vi "interface.vi"() -> ()   [LabVIEW 2019]
panel:
  out "alerte  2":bool=TRUE
  out "Error out 2":errorcluster
  out "marches _2":bool
  out "marche_one":bool
  out "alerte_high":bool
  out "alerte":bool
  out "type_sel":string
  out "concatenated string":string
  out ".not. x?":bool
  out "error out 4":errorcluster
  out "Error out":errorcluster
  in  "Add Square":bool
  in  "Database Square":bool
  in  "Dashboard Square":bool
  in  "Settings Square":bool
  in  "Tools Square":bool
  in  "Log Out Square":bool
  out "Log In Square":bool
  in  "Tab Control":enum32{"Page 1", "Page 2"}(tab)
  out "rouge":bool
  out "orange":bool
  out "vert":bool
  out "Historique des alertes":string
  in  "Tab Control 2":T1(tab)
  out "Boolean":bool
  in  "password":string
  in  "user name":string
  in  "Login Button":bool
  in  "Information Button":bool
  in  "type maintenace":bool
  in  "Energy 2":bool
  in  "Database Button":bool
  in  "Energy":bool
  in  "comp_2":bool
  in  "comp_1":bool
  in  "Tools Button":bool
  in  "autre maintenance":bool
  in  "Back Button":bool
  in  "compresseur id":dbl
  in  "Cluster 2":T2
  in  "Cluster":T3
  out "Derniére date de changement  H":string
  out "Nombre d'heure de marche H":string
  out "Durée de vie du huile":string
  out "Derniére date de changement C":string
  out "Nombre d'heure de marche C":string
  out "Durée de vie du courroie":string
  in  "autre maintenace bouton":bool
  in  "retour autre maintenace":bool
  in  "ID Comp":dbl
  in  "Commantaire":string
  in  "Description":string(combo)
  in  "Type maintenace":string(combo)
  out "error out 3":errorcluster
  in  "Back Square":bool
  out "error out 2":errorcluster
  in  "Url":string(combo)
  in  "Nom de la base":string(combo)
  in  "Back from 1":bool
  out "Debit":i32(knob) caption="Gauge" scale=0.0..80.0
  out "Etat":string
  out "Graphe de pression":cluster{timestamp[], dbl[]}(graph) caption="XY Graph - Dark"
  out "Graphe de Température":cluster{timestamp[], dbl[]}(graph) caption="XY Graph - Dark"
  out "Courant":i32(knob) caption="Gauge" scale=0.0..150.0
  out "Tension":i32(knob) caption="Gauge" scale=0.0..450.0
  out "Pression":i32(knob) caption="Gauge" scale=0.0..15.0
  out "Température":i32(knob) caption="Gauge" scale=0.0..150.0
  in  "Back from 2":bool
  out "Graphe de pression  2":cluster{timestamp[], dbl[]}(graph) caption="XY Graph - Dark"
  out "Graphe de Température":cluster{timestamp[], dbl[]}(graph) caption="XY Graph - Dark"
  out "Debit":i32(knob) caption="Gauge" scale=0.0..50.0
  out "Etat 2":string
  out "Courant  2":i32(knob) caption="Gauge" scale=0.0..150.0
  out "Tension 2":i32(knob) caption="Gauge" scale=0.0..250.0
  out "Pression 2":i32(knob) caption="Gauge" scale=0.0..10.0
  out "Température  2":i32(knob) caption="Gauge" scale=0.0..150.0
  out "COUT EN DT":dbl format="%_10g"
  in  "Prix KWH":string(combo)
  in  "Back from 3":bool
  in  "ID compresseur":dbl
  out "temp de marche en heure":dbl
  out "energie consommer kwh":dbl format="%_11g"
  in  "Date Fin":timestamp format="%<%.0X %x>T"
  in  "Date Debut":timestamp format="%<%.0X %x>T"
  out "Taux d’utilisation (%)":string
  out "Pression moyenne":string
  out "température moyenne":string
  out "Temps d'arret total":string
  in  "Back from 4":bool
  in  "ID compresseur":dbl
  out "Temps de fonctionnement total":string
  out "Nombre de démarrages / arrêts":string
  in  "Date Fin":timestamp format="%<%.0X %x>T"
  in  "Date Debut":timestamp format="%<%.0X %x>T"
  in  "Back Button 3":bool
  out "Historique des maintenances":string[][](table)
  out "Historique des alertes":string[][](table)
  in  "Back Button 4":bool
  in  "Add Button":bool
  in  "Role":string(combo)
  in  "Email":string
  in  "Mot de passe":string
  in  "Nom utilisateur":string
  in  "Back Button 2":bool
  in  "suivent":bool
  in  "TYPE C":bool
  in  "TYPE B":bool
  in  "type A":bool
  in  "Tab Control 3":enum32{"Page 1", "Page 2", "Page 3"}(tab)
  out "Nombre d'heures":dbl(slide)=1.0 scale=0.0..500.0
  out "Temps restants A":string
  out "Nombre d'heures":dbl(slide)=1.0 scale=0.0..1000.0
  out "Temps restants B":string
  out "Nombre d'heures":dbl(slide)=1.0 scale=0.0..4000.0
  out "Temps restants C":string
  in  "Temps de la maintenace":timestamp format="%<%H:%M>T"
  in  "Back Button 5":bool
  in  "Save Button":bool
  in  "Remarque":string
  in  "taches_principales":string
  in  "type_description":string(combo)
  in  "Type Maintenance":string(combo)
  out "Cluster - Thin Border 2":T4
  out "Cluster - Thin Border":T4
  in  "Back Button 6":bool
  # "Menu principale"
  # "Autre Maintenance"
  # "Paramètres"
  # "Controle énergie"
  # "kpi Performance"
  # "Historique"
  # "ajouter user"
  # "Maintenance type A :"
  # "Maintenance légère (préventive rapide)\nTâches à réaliser :\n\n-Vérification visuelle générale de la machine (fuites d’air, bruits anormaux).\n-Contrôle du niveau et de la qualité de l’huile.\n-Vidange de l’huile (si nécessaire selon le type d’huile).\n-Nettoyage des filtres d’aspiration d’air.\n-Inpection des courroies (tension et usure).\n-Contrôle de la température de fonctionnement.\n-Vérification des voyants d’alerte ou codes erreurs sur le pupitre."
  # "Maintenance type B :"
  # "Maintenance intermédiaire (préventive approfondie)\nTâches à réaliser :\n\n-Remplacement des courroies (même si elles ne semblent pas endommagées).\n-Remplacement systématique de l’huile du compresseur.\n-Nettoyage ou remplacement du filtre à air.\n-Nettoyage du refroidisseur (radiateur) pour éviter la surchauffe.\n-Vérification de la consommation électrique pour détecter les anomalies.\n-Contrôle du moteur électrique (bruit, vibrations, température)."
  # "Maintenance type C :"
  # "Maintenance lourde (grande révision)\nTâches à réaliser :\n\n-Remplacement des roulements du moteur et du compresseur.\n-Contrôle précis de l’étanchéité de tout le circuit d’air.\n-Recalibrage des capteurs de pression et de température.\n-Contrôle des soupapes (entrée/sortie) et nettoyage ou remplacement.\n-Inspection complète de la vis de compression (si applicable)."
  # "Info"
  # "Champ                                                           Valeur"
  # "Champ                                                           Valeur"
types:
  T1 = enum32{"Page 1", "Page 2", "Page 3", "Page 4", "Page 5", "Page 6", "Page 7", "Page 8", "Page 11", "Page 9", "Page 10", "Page 12", "Page 13", "Page 14"}
  T2 = cluster{"Save Button":bool, "Durée de vie huile ":dbl, "Description ":string, "Commantaire":string}
  T3 = cluster{"Save Button":bool, "Durée de vie courroie ":dbl, "Description ":string, "Commantaire":string}
  T4 = cluster{"Nom du compresseur":string, "Numéro de série\t":string, "Modèle\t":string, "Date de mise en service\t":string, "État actuel\t":string, "Heures de fonctionnement\t":string}
  T5 = enum32{"Page 1", "Page 2", "Page 3", "Page 4", "Page 5", "Page 6", "Page 7", "Page 8", "Page 11", "Page 9", "Page 10"}
  T6 = enum8{"Enabled", "Disabled", "Disabled and Grayed Out"}
  T7 = enum32{"Page 1", "Page 2", "Page 3", "Page 4", "Page 5", "Page 6", "Page 7", "Page 8", "Page 11", "Page 9", "Page 10", "Page 12", "Page 13"}
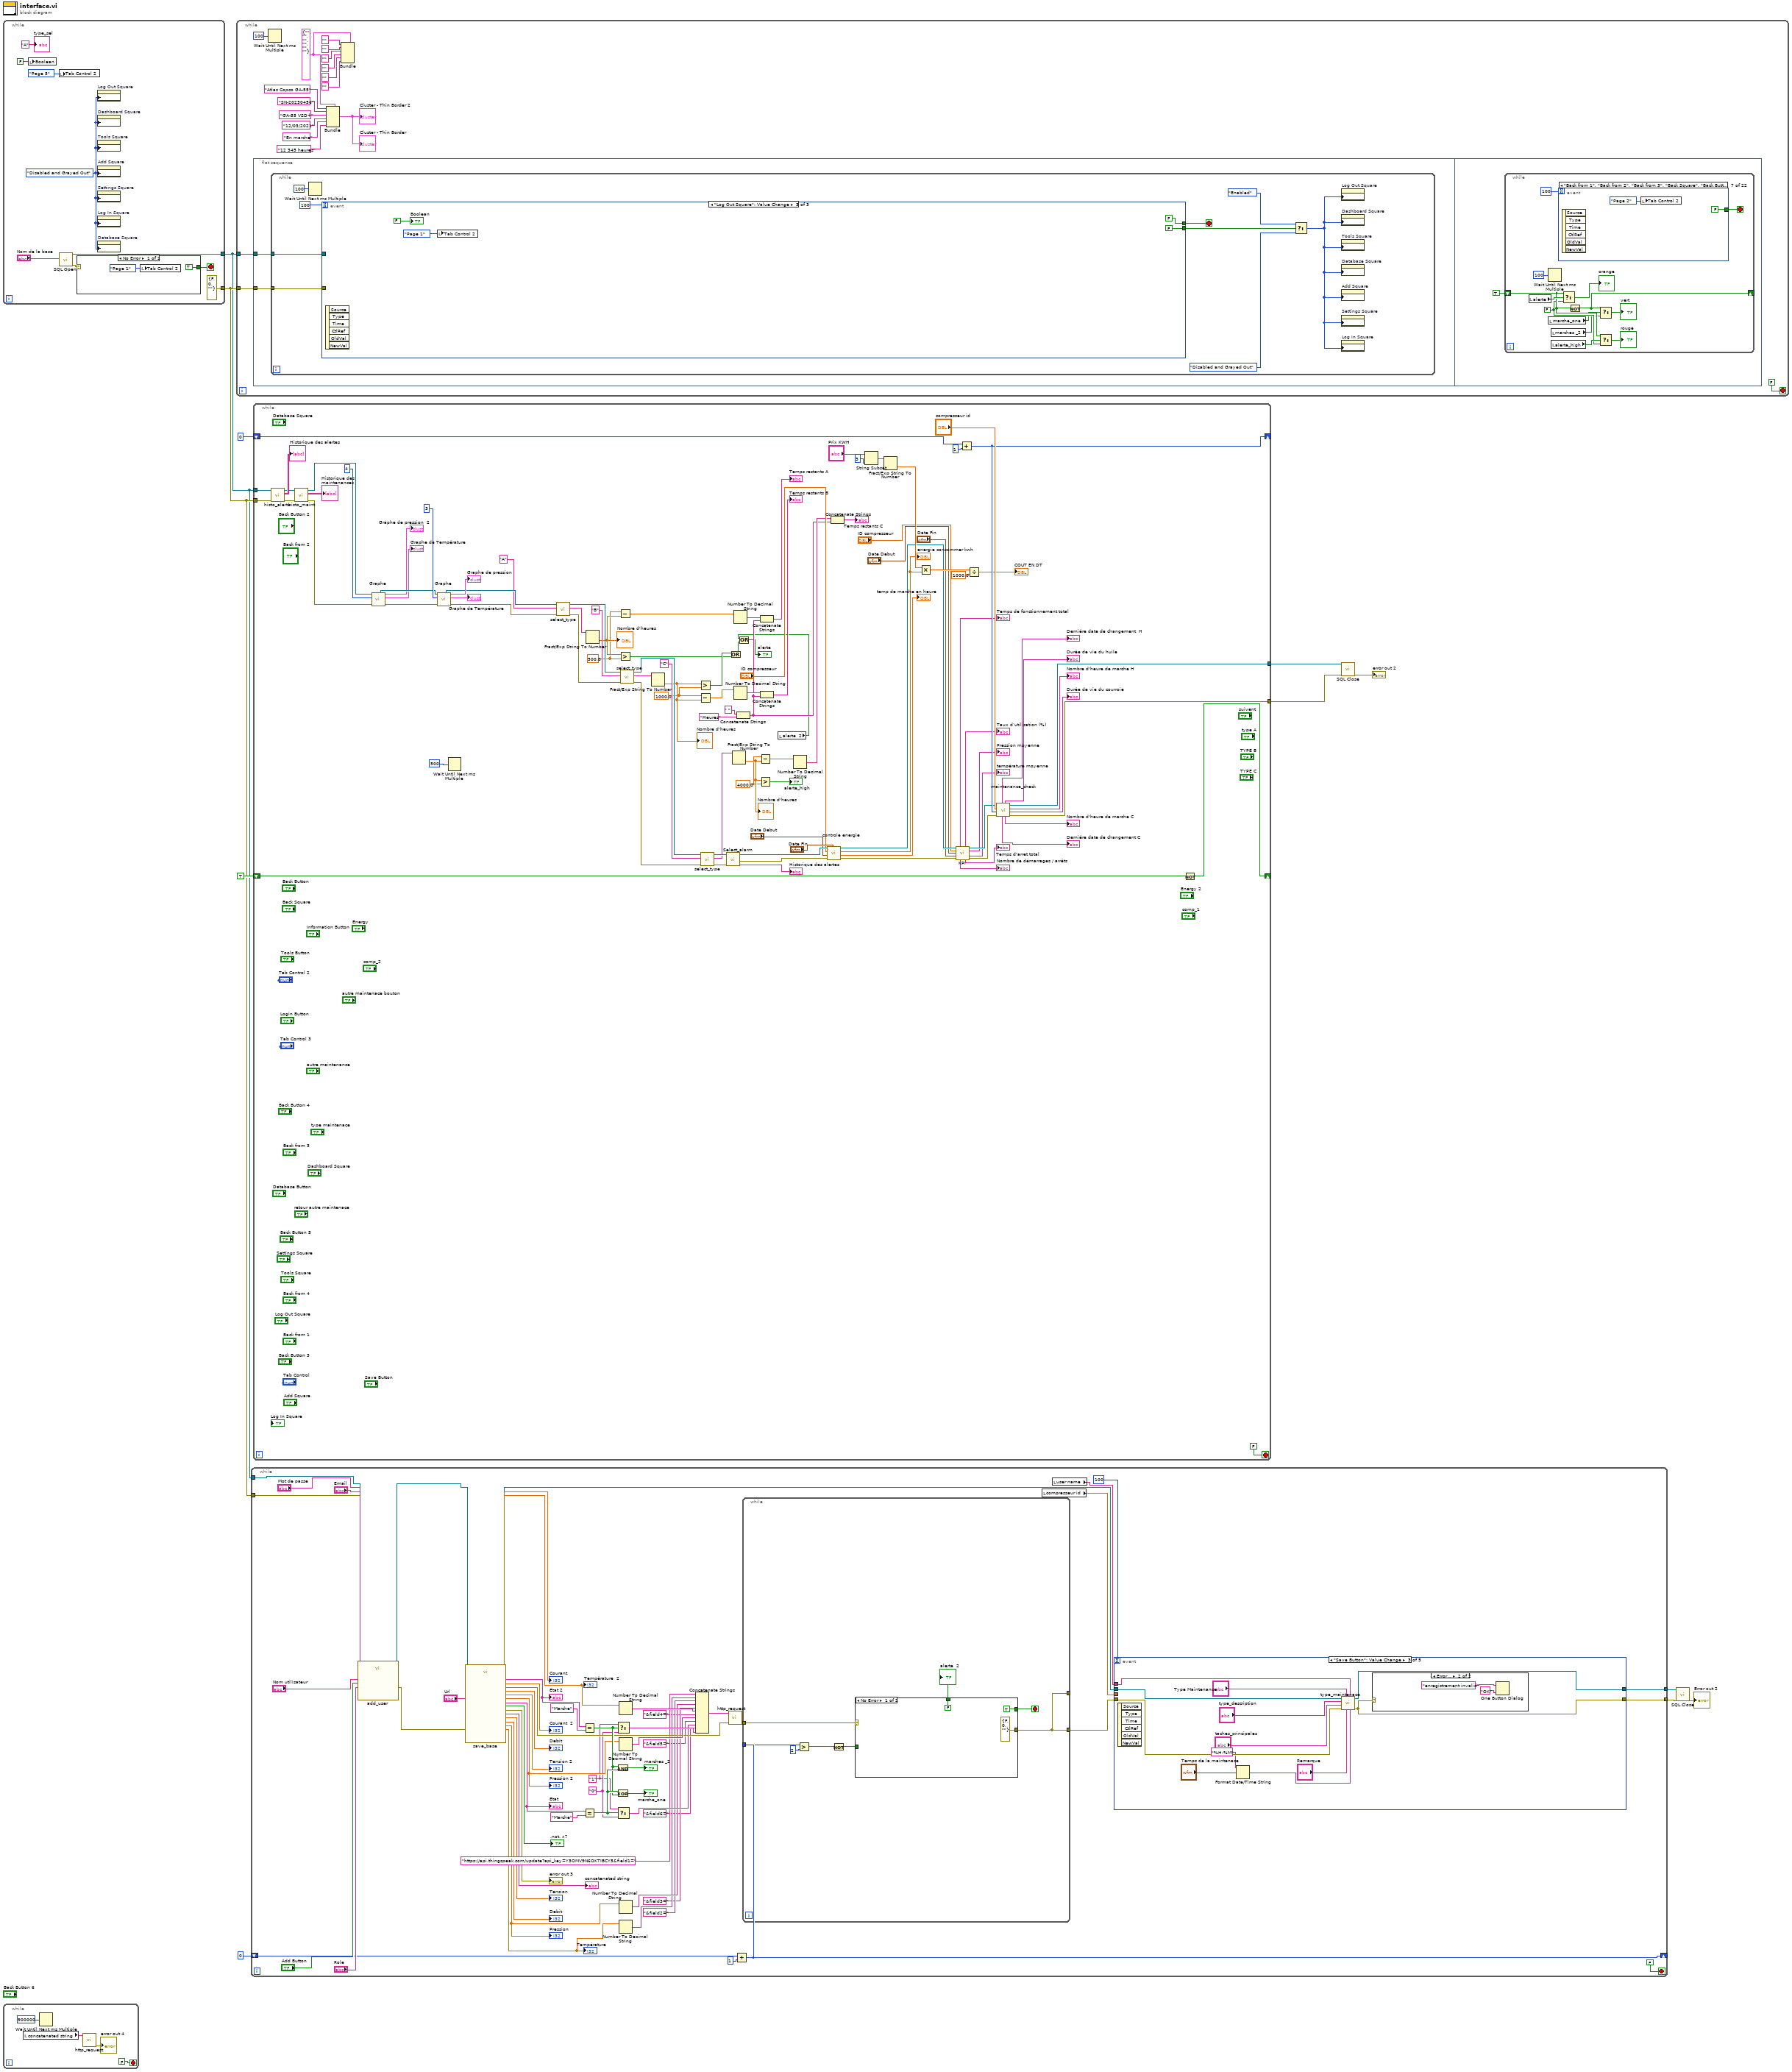
[diagram p0: block diagram]
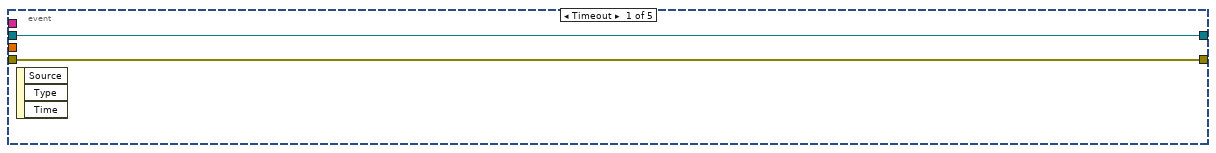
[diagram p2: hidden frame]
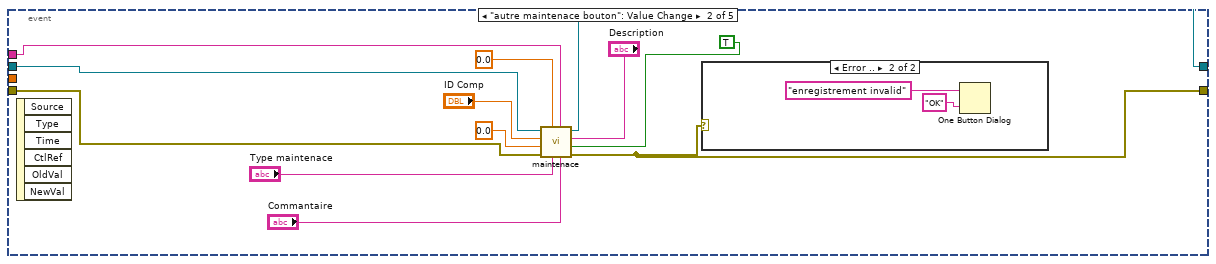
[diagram p3: hidden frame]
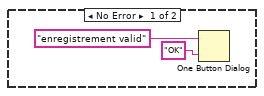
[diagram p4: hidden frame]
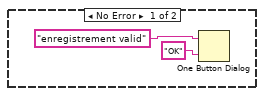
[diagram p5: hidden frame]
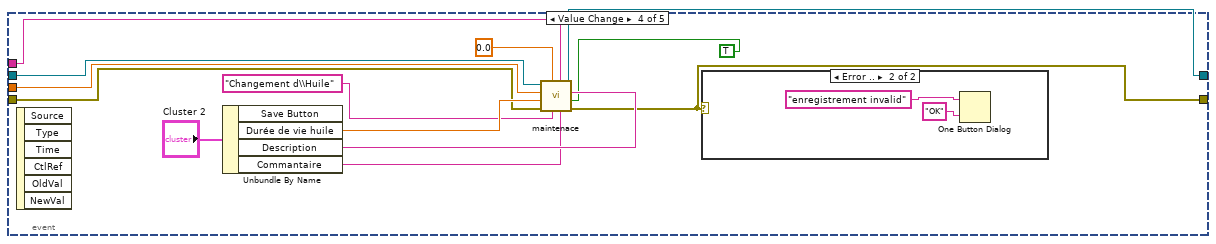
[diagram p6: hidden frame]
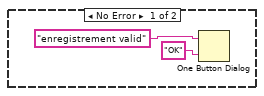
[diagram p7: hidden frame]
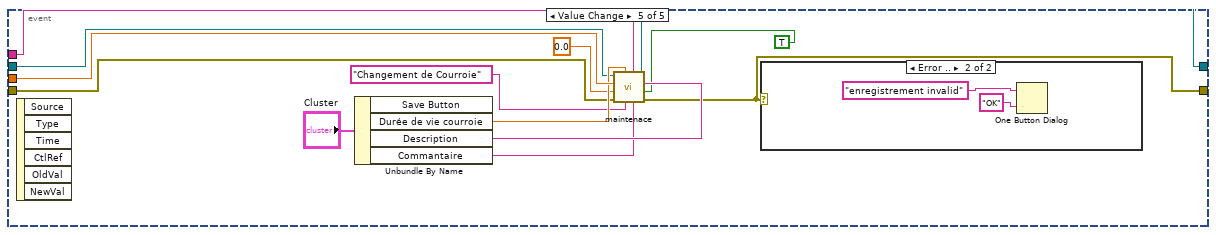
[diagram p8: hidden frame]
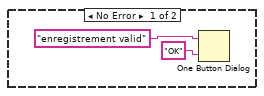
[diagram p9: hidden frame]
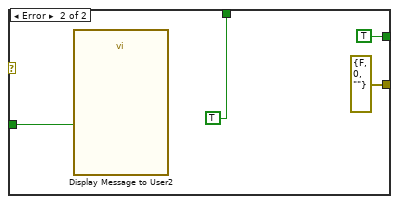
[diagram p10: hidden frame]
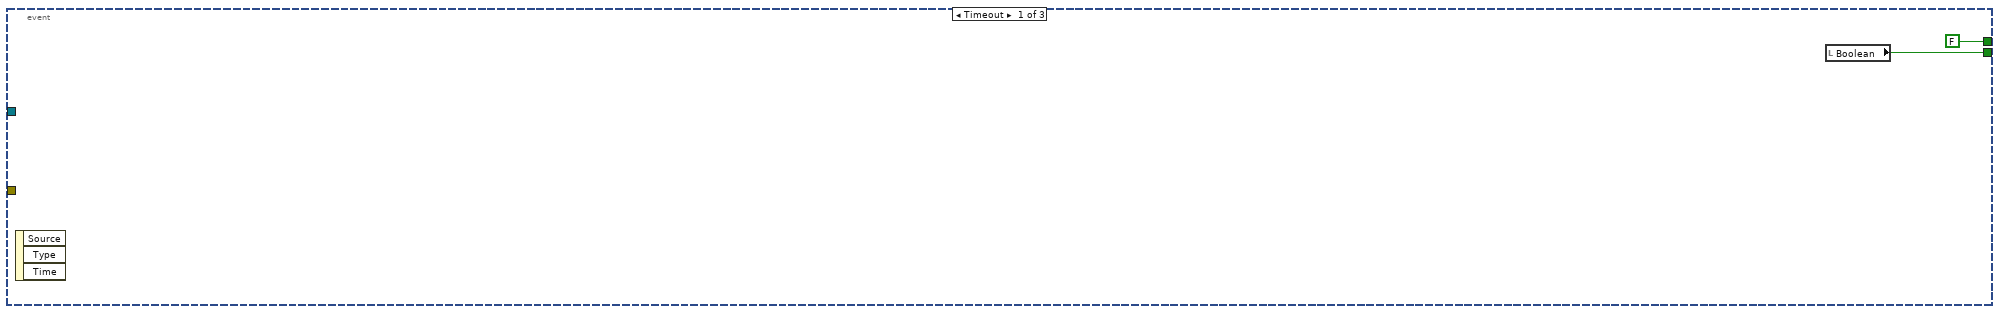
[diagram p11: hidden frame]
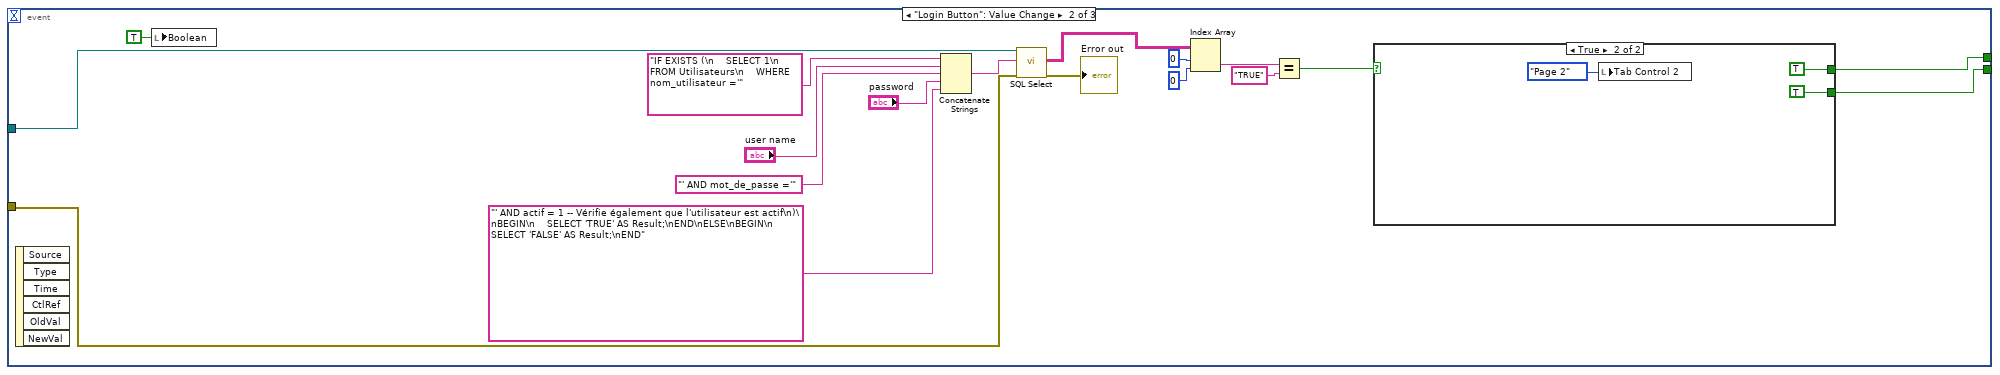
[diagram p12: hidden frame]
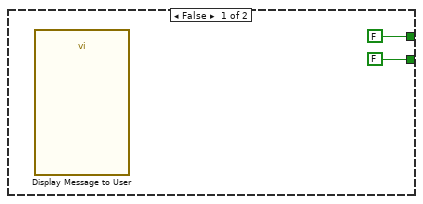
[diagram p13: hidden frame]
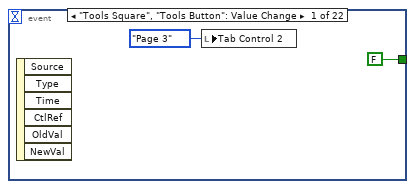
[diagram p14: hidden frame]
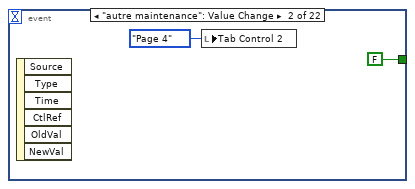
[diagram p15: hidden frame]
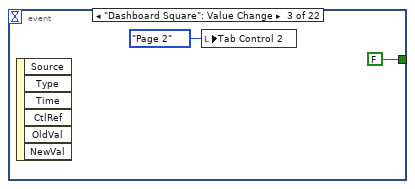
[diagram p16: hidden frame]
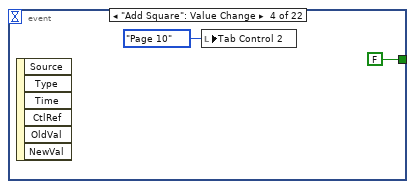
[diagram p17: hidden frame]
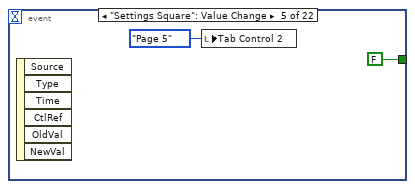
[diagram p18: hidden frame]
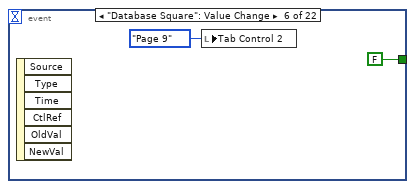
[diagram p19: hidden frame]
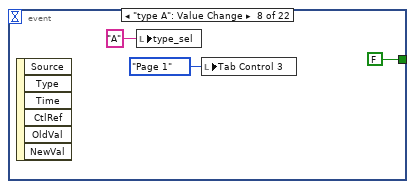
[diagram p20: hidden frame]
diagram:
  n1 = while {
    tunnel: [errorcluster {"status"=FALSE, "code"=0, "source"=""} ("Error out")] -> w6
    tunnel: [w20] -> w5
    stop <- w16 stop-if-true
    w13 = T6."Disabled and Grayed Out" ("Disabled")
    n2 = local write "Boolean"(FALSE ("Boolean")) -> ()
    n3 = local write "Tab Control 2"(T5."Page 5" ("Tab Control 2")) -> ()
    n4 = call <vilib>:"SQL Open.vi"("ConnectionString In"="Nom de la base") -> ("Connection Out"=w20:refnum<k7>, "Error out"=w17:errorcluster)  [unwired: 17 in]
    n5 = case shown="No Error" w17 {
      tunnel: [TRUE FALSE] -> w16
      frame No Error {
        n6 = local write "Tab Control 2"(enum32{"Page 1", "Page 2"}."Page 1" ("Tab Control 2")) -> ()
      }
      frame Error {
      }
    }
    n7 = property on="Log Out Square" class="Bool"("DisabledEnum"=w13) -> ()  [unwired: 2 in, 2 out]
    n8 = property on="Dashboard Square" class="Bool"("DisabledEnum"=w13) -> ()  [unwired: 2 in, 2 out]
    n9 = property on="Tools Square" class="Bool"("DisabledEnum"=w13) -> ()  [unwired: 2 in, 2 out]
    n10 = property on="Add Square" class="Bool"("DisabledEnum"=w13) -> ()  [unwired: 2 in, 2 out]
    n11 = property on="Settings Square" class="Bool"("DisabledEnum"=w13) -> ()  [unwired: 2 in, 2 out]
    n12 = property on="Log In Square" class="Bool"("DisabledEnum"=w13) -> ()  [unwired: 2 in, 2 out]
    n13 = property on="Database Square" class="Bool"("DisabledEnum"=w13) -> ()  [unwired: 2 in, 2 out]
    "type_sel" <- "A"
  }
  n14 = while {
    stop <- FALSE stop-if-true
    n15 = local read "concatenated string"() -> (w24:string)
    n16 = Wait Until Next ms Multiple(millisecond multiple=u32 900000) -> ()  [unwired: 1 out]
    n17 = call "http_request.vi"("url"=w24) -> ("error out"=→"error out 4":errorcluster)  [unwired: 10 in]
  }
  n18 = while {
    tunnel: w5 -> [w45]
    tunnel: w6 -> [w44]
    stop <- FALSE stop-if-true
    w41 = T4 {"Nom du compresseur"="", "Numéro de série\t"="", "Modèle\t"="", "Date de mise en service\t"="", "État actuel\t"="", "Heures de fonctionnement\t"=""} ("Cluster - Thin Border")
    n19 = flat-sequence {
      tunnel: w45 -> [w47]
      tunnel: w44 -> [w46]
      frame #0 {
        n20 = while {
          tunnel: w47 -> [w56]
          tunnel: w46 -> [w55]
          stop <- w48 stop-if-true
          n21 = Wait Until Next ms Multiple(millisecond multiple=u32 100) -> ()  [unwired: 1 out]
          n22 = event shown="[2] \"Log Out Square\": Value Change" {
            selector: _ -> [_ _ _]
            dyn-events: _ -> [_ _ _]
            timeout: 100 -> [_ _ _]
            tunnel: [w57 w76 FALSE] -> w49
            tunnel: w56 -> [_ w63 _]
            tunnel: w55 -> [_ w62 _]
            tunnel: [FALSE w61 FALSE] -> w48
            event Timeout {
              n23 = event-data() -> ()  [unwired: 1 in, 3 out]
              n24 = local read "Boolean"() -> (w57:bool)
            }
            event "Login Button": Value Change {
              n25 = event-data() -> ()  [unwired: 1 in, 6 out]
              n26 = local write "Boolean"(TRUE ("Boolean")) -> ()
              n27 = Concatenate Strings("IF EXISTS (\n    SELECT 1\n    FROM Utilisateurs\n    WHERE nom_utilisateur ='" ("string"), "user name", "' AND mot_de_passe ='" ("string"), "password", "' AND actif = 1 -- Vérifie également que l'utilisateur est actif\n)\nBEGIN\n    SELECT 'TRUE' AS Result;\nEND\nELSE\nBEGIN\n    SELECT 'FALSE' AS Result;\nEND" ("SQL Query")) -> (w72:string)
              n28 = call <vilib>:"SQL Select.vi"("Connection In"=w63, "SQL Query"=w72, "Error in (no error)"=w62) -> ("Data"=w69:string[][], "Error out"=→"Error out":errorcluster)  [unwired: 14 in, 1 out]
              n29 = Index Array(array=w69, index (row)=0, index (col)=0 ("disabled index (col)")) -> (element=w66:string)
              n30 = Equal?(x=w66, y="TRUE") -> (x = y?=w65:bool)
              n31 = case shown="True" w65 {
                tunnel: [FALSE TRUE] -> w76
                tunnel: [FALSE TRUE] -> w61
                frame False {
                  n32 = call "Display Message to User"() -> ()  [unwired: 10 in, 2 out]
                }
                frame True {
                  n33 = local write "Tab Control 2"(enum32{"Page 1", "Page 2"}."Page 2" ("Tab Control 2")) -> ()
                }
              }
            }
            event "Log Out Square": Value Change {
              n34 = event-data() -> ()  [unwired: 1 in, 6 out]
              n35 = local write "Tab Control 2"(enum32{"Page 1", "Page 2"}."Page 1" ("Tab Control 2")) -> ()
              "Boolean" <- FALSE ("Boolean")
            }
          }
          n36 = Select(t=T6."Enabled" ("Disabled"), s=w49, f=T6."Disabled and Grayed Out" ("Disabled")) -> (s? t:f=w52:T6)
          n37 = property on="Log Out Square" class="Bool"("DisabledEnum"=w52) -> ()  [unwired: 2 in, 2 out]
          n38 = property on="Dashboard Square" class="Bool"("DisabledEnum"=w52) -> ()  [unwired: 2 in, 2 out]
          n39 = property on="Tools Square" class="Bool"("DisabledEnum"=w52) -> ()  [unwired: 2 in, 2 out]
          n40 = property on="Database Square" class="Bool"("DisabledEnum"=w52) -> ()  [unwired: 2 in, 2 out]
          n41 = property on="Add Square" class="Bool"("DisabledEnum"=w52) -> ()  [unwired: 2 in, 2 out]
          n42 = property on="Settings Square" class="Bool"("DisabledEnum"=w52) -> ()  [unwired: 2 in, 2 out]
          n43 = property on="Log In Square" class="Bool"("DisabledEnum"=w52) -> ()  [unwired: 2 in, 2 out]
        }
      }
      frame #1 {
        n44 = while {
          shift-right: [w88] -> _
          shift-left: TRUE -> [w93]
          stop <- w98 stop-if-true
          w92 = FALSE ("f")
          n45 = local read "alerte"() -> (w96:bool)
          n46 = Wait Until Next ms Multiple(millisecond multiple=u32 100) -> ()  [unwired: 1 out]
          n47 = local read "marche_one"() -> (w89:bool)
          n48 = local read "marches _2"() -> (w87:bool)
          n49 = local read "alerte_high"() -> (w94:bool)
          n50 = event shown="[6] \"Back from 1\", \"Back from 2\", \"Back from 3\", \"Back Square\", \"Back Button 3\", \"Back Button 4\", \"Back from 4\", \"Back Button 2\", \"Back Button 6\": Value Change" {
            selector: _ -> [_ _ _ _ _ _ _ _ _ _ _ _ _ _ _ _ _ _ _ _ _ _]
            dyn-events: _ -> [_ _ _ _ _ _ _ _ _ _ _ _ _ _ _ _ _ _ _ _ _ _]
            timeout: 100 -> [_ _ _ _ _ _ _ _ _ _ _ _ _ _ _ _ _ _ _ _ _ _]
            tunnel: [FALSE FALSE FALSE FALSE FALSE FALSE FALSE FALSE FALSE FALSE FALSE FALSE FALSE FALSE FALSE TRUE FALSE FALSE FALSE FALSE FALSE FALSE] -> w98
            event "Tools Square", "Tools Button": Value Change {
              n51 = event-data() -> ()  [unwired: 1 in, 6 out]
              n52 = local write "Tab Control 2"(T5."Page 3" ("Tab Control 2")) -> ()
            }
            event "autre maintenance": Value Change {
              n53 = event-data() -> ()  [unwired: 1 in, 6 out]
              n54 = local write "Tab Control 2"(T5."Page 4" ("Tab Control 2")) -> ()
            }
            event "Dashboard Square": Value Change {
              n55 = event-data() -> ()  [unwired: 1 in, 6 out]
              n56 = local write "Tab Control 2"(T5."Page 2" ("Tab Control 2")) -> ()
            }
            event "Add Square": Value Change {
              n57 = event-data() -> ()  [unwired: 1 in, 6 out]
              n58 = local write "Tab Control 2"(T5."Page 10" ("Tab Control 2")) -> ()
            }
            event "Settings Square": Value Change {
              n59 = event-data() -> ()  [unwired: 1 in, 6 out]
              n60 = local write "Tab Control 2"(T5."Page 5" ("Tab Control 2")) -> ()
            }
            event "Database Square": Value Change {
              n61 = event-data() -> ()  [unwired: 1 in, 6 out]
              n62 = local write "Tab Control 2"(T5."Page 9" ("Tab Control 2")) -> ()
            }
            event "Back from 1", "Back from 2", "Back from 3", "Back Square", "Back Button 3", "Back Button 4", "Back from 4", "Back Button 2", "Back Button 6": Value Change {
              n63 = event-data() -> ()  [unwired: 1 in, 6 out]
              n64 = local write "Tab Control 2"(T5."Page 2" ("Tab Control 2")) -> ()
            }
            event "type A": Value Change {
              n65 = event-data() -> ()  [unwired: 1 in, 6 out]
              n66 = local write "type_sel"("A" ("type_sel")) -> ()
              n67 = local write "Tab Control 3"(enum32{"Page 1", "Page 2", "Page 3"}."Page 1" ("Tab Control 3")) -> ()
            }
            event "TYPE B": Value Change {
              n68 = event-data() -> ()  [unwired: 1 in, 6 out]
              n69 = local write "type_sel"("B" ("type_sel")) -> ()
              n70 = local write "Tab Control 3"(enum32{"Page 1", "Page 2", "Page 3"}."Page 2" ("Tab Control 3")) -> ()
            }
            event "TYPE C": Value Change {
              n71 = event-data() -> ()  [unwired: 1 in, 6 out]
              n72 = local write "type_sel"("C" ("type_sel")) -> ()
              n73 = local write "Tab Control 3"(enum32{"Page 1", "Page 2", "Page 3"}."Page 3" ("Tab Control 3")) -> ()
            }
            event "comp_1": Value Change {
              n74 = event-data() -> ()  [unwired: 1 in, 6 out]
              n75 = local write "Tab Control 2"(T5."Page 6" ("Tab Control 2")) -> ()
            }
            event "comp_2": Value Change {
              n76 = event-data() -> ()  [unwired: 1 in, 6 out]
              n77 = local write "Tab Control 2"(T5."Page 7" ("Tab Control 2")) -> ()
            }
            event "Back Button": Value Change {
              n78 = event-data() -> ()  [unwired: 1 in, 6 out]
              n79 = local write "Tab Control 2"(enum32{"Page 1", "Page 2"}."Page 2" ("Tab Control 2")) -> ()
            }
            event "Energy": Value Change {
              n80 = event-data() -> ()  [unwired: 1 in, 6 out]
              n81 = local write "Tab Control 2"(T5."Page 8" ("Tab Control 2")) -> ()
            }
            event "Database Button": Value Change {
              n82 = event-data() -> ()  [unwired: 1 in, 6 out]
              n83 = local write "Tab Control 2"(T5."Page 9" ("Tab Control 2")) -> ()
            }
            event "Log Out Square": Value Change {
              n84 = event-data() -> ()  [unwired: 1 in, 6 out]
              n85 = local write "Tab Control 2"(T5."Page 1" ("Tab Control 2")) -> ()
            }
            event "suivent": Value Change {
              n86 = event-data() -> ()  [unwired: 1 in, 6 out]
              n87 = local write "Tab Control 2"(T7."Page 13" ("Tab Control 2")) -> ()
            }
            event "type maintenace", "Back Button 5": Value Change {
              n88 = event-data() -> ()  [unwired: 1 in, 6 out]
              n89 = local write "Tab Control 2"(T7."Page 12" ("Tab Control 2")) -> ()
            }
            event "Information Button": Value Change {
              n90 = event-data() -> ()  [unwired: 1 in, 6 out]
              n91 = local write "Tab Control 2"(T1."Page 14" ("Tab Control 2")) -> ()
            }
            event "Energy 2": Value Change {
              n92 = event-data() -> ()  [unwired: 1 in, 6 out]
              n93 = local write "Tab Control 2"(T5."Page 11" ("Tab Control 2")) -> ()
            }
            event Timeout {
              n94 = event-data() -> ()  [unwired: 1 in, 3 out]
            }
            event "retour autre maintenace": Value Change {
              n95 = event-data() -> ()  [unwired: 1 in, 6 out]
              n96 = local write "Tab Control 2"(T5."Page 3" ("Tab Control 2")) -> ()
            }
          }
          n97 = Select(t=w93, s=w96, f=w92) -> (s? t:f=→"orange":bool)
          n98 = Not(x=w93) -> (.not. x?=w88:bool)
          n99 = Select(t=w88, s=w89, f=w87) -> (s? t:f=→"vert":bool)
          n100 = Select(t=w93, s=w94, f=w92) -> (s? t:f=→"rouge":bool)
        }
      }
    }
    n101 = Wait Until Next ms Multiple(millisecond multiple=u32 100) -> ()  [unwired: 1 out]
    n102 = Bundle(cluster=w41, "Nom du compresseur"="Atlas Copco GA-55", "Numéro de série"="SN-20230456", "Modèle"="GA-55 VSD+", "Date de mise en service"="12/03/2021", "État actuel"="En marche", "Heures de fonctionnement"="12 345 heures") -> (→"Cluster - Thin Border 2" →"Cluster - Thin Border":T4)
    n103 = Bundle(cluster=w41, "Nom du compresseur"="", "Numéro de série"="", "Modèle"="", "Date de mise en service"="", "État actuel"="", "Heures de fonctionnement"="") -> ()  [unwired: 1 out]
  }
  n104 = while {
    tunnel: w6 -> [w158]
    tunnel: w5 -> [w157]
    tunnel: [w150] -> w4
    tunnel: [w149] -> w3
    shift-right: [w146] -> _
    shift-left: 0 -> [w147]
    stop <- FALSE stop-if-true
    w169 = "0" ("f")
    w168 = "1"
    n105 = call "add_user.vi"("Add Button"="Add Button", "Nom utilisateur"="Nom utilisateur", "Role"="Role", "Error out"=w158, "Email"="Email", "Mot de passe"="Mot de passe", "Connection in"=w157) -> ("Error out 2"=w159:errorcluster, "Connection Out 2"=w156:refnum<k7>)  [unwired: 3 in]
    n106 = call "save_base.vi"("Connection In"=w156, "Url"="Url", "Error in (no error)"=w159) -> ("concatenated string"=→"concatenated string":string, "error out"=→"error out 3":errorcluster, ".not. x?"=→".not. x?":bool, "Tension"=→"Tension":dbl, "Etat"=w194:string, "Debit"=→"Debit":dbl, "Pression 2"=w186:dbl, "Pression"=w183:dbl, "Tension2"=→"Tension 2":dbl, "temperature"=w178:dbl, "Debit  2"=→"Debit":dbl, "Connection Out"=w151:refnum<k7>, "Courant"=→"Courant":dbl, "temperature 2"=w185:dbl, "etat 2"=w190:string, "Courant 2"=→"Courant  2":dbl, "Error out"=w181:errorcluster)
    "Température" <- w178
    "Pression" <- w183
    "Etat" <- w194
    "Pression 2" <- w186
    "Etat 2" <- w190
    "Température  2" <- w185
    n107 = Equal?(x=w190, y="Marche") -> (x = y?=w195:bool)
    n108 = Equal?(x=w194, y="Marche") -> (x = y?=w196:bool)
    n109 = And(x=w195, y=w196) -> (x .and. y?=→"marches _2":bool)
    n110 = Exclusive Or(1:w195, 2:w196) -> (0:→"marche_one":bool)
    n111 = Select(t=w168, s=w195, f=w169) -> (s? t:f=w191:string)
    n112 = Select(t=w168, s=w196, f=w169) -> (s? t:f=w189:string)
    n113 = Number To Decimal String(number=w185) -> (decimal integer string=w187:string)  [unwired: 1 in]
    n114 = Number To Decimal String(number=w186) -> (decimal integer string=w188:string)  [unwired: 1 in]
    n115 = Number To Decimal String(number=w183) -> (decimal integer string=w184:string)  [unwired: 1 in]
    n116 = Number To Decimal String(number=w178) -> (decimal integer string=w180:string)  [unwired: 1 in]
    n117 = Concatenate Strings("https://api.thingspeak.com/update?api_key=Y3OMV9N6OKTIBCY5&field1=" ("string"), w180, "&field2=" ("string"), w184, "&field3=" ("string"), w187, "&field4=" ("string"), w188, "&field5=" ("string"), w189, "&field6=" ("string"), w191) -> (w179:string)
    n118 = call "http_request.vi"("error in (no error)"=w181, "url"=w179) -> ("error out"=w182:errorcluster)  [unwired: 9 in]
    n119 = Add(x=w147, y=1) -> (x+y=w146:i32)
    n120 = while {
      tunnel: w182 -> [w279]
      tunnel: [w275] -> _
      tunnel: [w275] -> w152
      tunnel: w146 -> [w274]
      stop <- w280 stop-if-true
      n121 = Greater?(x=w274, y=2) -> (0:w277:bool)
      n122 = Not(x=w277) -> (.not. x?=w276:bool)
      n123 = case shown="No Error" w279 {
        tunnel: [errorcluster {"status"=FALSE, "code"=0, "source"=""} ("Error in (no error)") errorcluster {"status"=FALSE, "code"=0, "source"=""} ("Error in (no error)")] -> w275
        tunnel: [TRUE ("true") TRUE ("true")] -> w280
        tunnel: w276 -> [_ w286]
        tunnel: [FALSE ("alerte") TRUE ("alerte")] -> w273
        frame No Error {
        }
        frame Error {
          n124 = call "Display Message to User2"("Enable"=w286) -> ()  [unwired: 9 in, 2 out]
        }
      }
      "alerte  2" <- w273
    }
    n125 = local read "compresseur id"() -> (w155:dbl)
    n126 = local read "user name"() -> (w154:string)
    n127 = event shown="[2] \"Save Button\": Value Change" {
      selector: _ -> [_ _ _ _ _]
      dyn-events: _ -> [_ _ _ _ _]
      timeout: 100 -> [_ _ _ _ _]
      tunnel: w154 -> [_ w210 w227 w251 w268]
      tunnel: w155 -> [_ _ _ w250 w267]
      tunnel: w151 -> [w206 w218 w234 w246 w260]
      tunnel: [w206 w217 w232 w245 w259] -> w150
      tunnel: w152 -> [w205 w208 w233 w244 w258]
      tunnel: [w205 w207 w226 w239 w256] -> w149
      event Timeout {
        n128 = event-data() -> ()  [unwired: 1 in, 3 out]
      }
      event "autre maintenace bouton": Value Change {
        n129 = event-data() -> ()  [unwired: 1 in, 6 out]
        n130 = call "maintenace.vi"("valid"=TRUE, "Description"="Description", "Commantaire"="Commantaire", "Non_technicien"=w210, "Type maintenance"="Type maintenace", "Durée_courroie"=0.0, "Error in (no error)"=w208, "durée_huile"=0.0, "id"="ID Comp", "Connection In"=w218) -> ("Error out"=w207:errorcluster, "Connection Out"=w217:refnum<k7>)
        n131 = case shown="Error .." w207 {
          frame No Error {
            n132 = One Button Dialog(message="enregistrement valid", button name ("OK")="OK") -> ()  [unwired: 1 out]
          }
          frame Error {
            n133 = One Button Dialog(message="enregistrement invalid", button name ("OK")="OK") -> ()  [unwired: 1 out]
          }
        }
      }
      event "Save Button": Value Change {
        n134 = event-data() -> ()  [unwired: 1 in, 6 out]
        n135 = Format Date/Time String(time format string (%c)="%H:%M", seconds (now)="Temps de la maintenace") -> (date/time string=w223:string)  [unwired: 1 in]
        n136 = call "type_maintenace.vi"("durée"=w223, "technicien"=w227, "Remarque"="Remarque", "type"="Type Maintenance", "Error in (no error)"=w233, "taches_principales"="taches_principales", "type_description"="type_description", "Connection In"=w234) -> ("Error out"=w226:errorcluster, "Connection Out"=w232:refnum<k7>)  [unwired: 2 in]
        n137 = case shown="Error .." w226 {
          frame No Error {
            n138 = One Button Dialog(message="enregistrement valid", button name ("OK")="OK") -> ()  [unwired: 1 out]
          }
          frame Error {
            n139 = One Button Dialog(message="enregistrement invalid", button name ("OK")="OK") -> ()  [unwired: 1 out]
          }
        }
      }
      event "Cluster 2.Save Button": Value Change {
        n140 = event-data() -> ()  [unwired: 1 in, 6 out]
        n141 = Unbundle By Name("Cluster 2") -> ("Durée de vie huile"=w248:dbl, "Description"=w243:string, "Commantaire"=w242:string)  [unwired: 1 out]
        n142 = call "maintenace.vi"("valid"=TRUE, "Description"=w243, "Commantaire"=w242, "Non_technicien"=w251, "Type maintenance"="Changement d\\Huile", "Durée_courroie"=0.0, "Error in (no error)"=w244, "durée_huile"=w248, "id"=w250, "Connection In"=w246) -> ("Error out"=w239:errorcluster, "Connection Out"=w245:refnum<k7>)
        n143 = case shown="Error .." w239 {
          frame No Error {
            n144 = One Button Dialog(message="enregistrement valid", button name ("OK")="OK") -> ()  [unwired: 1 out]
          }
          frame Error {
            n145 = One Button Dialog(message="enregistrement invalid", button name ("OK")="OK") -> ()  [unwired: 1 out]
          }
        }
      }
      event "Cluster.Save Button": Value Change {
        n146 = event-data() -> ()  [unwired: 1 in, 6 out]
        n147 = Unbundle By Name("Cluster") -> ("Durée de vie courroie"=w265:dbl, "Description"=w263:string, "Commantaire"=w262:string)  [unwired: 1 out]
        n148 = call "maintenace.vi"("valid"=TRUE, "Description"=w263, "Commantaire"=w262, "Non_technicien"=w268, "Type maintenance"="Changement de Courroie", "Durée_courroie"=w265, "Error in (no error)"=w258, "durée_huile"=0.0, "id"=w267, "Connection In"=w260) -> ("Error out"=w256:errorcluster, "Connection Out"=w259:refnum<k7>)
        n149 = case shown="Error .." w256 {
          frame No Error {
            n150 = One Button Dialog(message="enregistrement valid", button name ("OK")="OK") -> ()  [unwired: 1 out]
          }
          frame Error {
            n151 = One Button Dialog(message="enregistrement invalid", button name ("OK")="OK") -> ()  [unwired: 1 out]
          }
        }
      }
    }
  }
  n152 = while {
    tunnel: [w291] -> w11
    tunnel: [w292] -> w10
    shift-right: [w359] -> _
    shift-left: 0 -> [w361]
    tunnel: w5 -> [w296]
    tunnel: w6 -> [w295]
    shift-right: [w316] -> _
    shift-left: TRUE -> [w317]
    stop <- FALSE stop-if-true
    w306 = 4000.0 ("x")
    w309 = 1000.0 ("y")
    w308 = 500.0 ("y")
    n153 = call "histo_alerte.vi"("Error in (no error)"=w295, "Connection In"=w296) -> ("Error out"=w357:errorcluster, "Table"=→"Historique des alertes":string[][], "Connection Out"=w356:refnum<k7>)  [unwired: 7 in]
    n154 = call "histo_maint.vi"("Error in (no error)"=w357, "Connection In"=w356) -> ("Error out"=w293:errorcluster, "Table"=→"Historique des maintenances":string[][], "Connection Out"=w294:refnum<k7>)  [unwired: 7 in]
    n155 = call "Graphe.vi"("Error in (no error)"=w293, "number"=4, "Connection In"=w294) -> ("Error out"=w373:errorcluster, "Graphe de temperature"=→"Graphe de Température":cluster{timestamp[], dbl[]}, "graphe de pression"=→"Graphe de pression  2":cluster{timestamp[], dbl[]}, "Connection Out"=w374:refnum<k7>)  [unwired: 5 in]
    n156 = call "Graphe.vi"("Error in (no error)"=w373, "number"=3, "Connection In"=w374) -> ("Error out"=w328:errorcluster, "Graphe de temperature"=→"Graphe de Température":cluster{timestamp[], dbl[]}, "graphe de pression"=→"Graphe de pression":cluster{timestamp[], dbl[]}, "Connection Out"=w331:refnum<k7>)  [unwired: 5 in]
    n157 = Wait Until Next ms Multiple(millisecond multiple=u32 500) -> ()  [unwired: 1 out]
    n158 = call "select_type.vi"("Error in (no error)"=w328, "type"="A", "Connection In"=w331) -> ("Error out"=w327:errorcluster, "nombre d'heures"=w320:string, "Connection Out"=w330:refnum<k7>)  [unwired: 6 in]
    n159 = Fract/Exp String To Number(string=w320) -> (number=w314:dbl)  [unwired: 3 in, 1 out]
    "Nombre d'heures" <- w314
    n160 = Subtract(x=w308, y=w314) -> (x-y=w313:dbl)
    n161 = Greater?(x=w314, y=w308) -> (0:w318:bool)
    n162 = call "select_type.vi"("Error in (no error)"=w327, "type"="B", "Connection In"=w330) -> ("Error out"=w326:errorcluster, "nombre d'heures"=w322:string, "Connection Out"=w329:refnum<k7>)  [unwired: 6 in]
    n163 = Fract/Exp String To Number(string=w322) -> (number=w312:dbl)  [unwired: 3 in, 1 out]
    "Nombre d'heures" <- w312
    n164 = Greater?(x=w312, y=w309) -> (0:w319:bool)
    n165 = Subtract(x=w309, y=w312) -> (x-y=w311:dbl)
    n166 = call "select_type.vi"("Error in (no error)"=w326, "type"="C", "Connection In"=w329) -> ("Error out"=w332:errorcluster, "nombre d'heures"=w321:string, "Connection Out"=w333:refnum<k7>)  [unwired: 6 in]
    n167 = call "Select_alarm.vi"("Error in (no error)"=w332, "Connection In"=w333) -> ("Historique alerte"=→"Historique des alertes":string, "Error out"=w362:errorcluster, "Connection Out"=w381:refnum<k7>)  [unwired: 7 in]
    n168 = Or(x=w319, y=w318) -> (x .or. y?=w290:bool)
    n169 = Fract/Exp String To Number(string=w321) -> (number=w307:dbl)  [unwired: 3 in, 1 out]
    "Nombre d'heures" <- w307
    n170 = Number To Decimal String(number=w313) -> (decimal integer string=w303:string)  [unwired: 1 in]
    n171 = Number To Decimal String(number=w311) -> (decimal integer string=w302:string)  [unwired: 1 in]
    n172 = Concatenate Strings(" " ("string"), "Heures") -> (w298:string)
    n173 = Subtract(x=w306, y=w307) -> (x-y=w310:dbl)
    n174 = Greater?(x=w307, y=w306) -> (0:→"alerte_high":bool)
    n175 = Concatenate Strings(w303, w298) -> (→"Temps restants A":string)
    n176 = Concatenate Strings(w302, w298) -> (→"Temps restants B":string)
    n177 = local read "alerte  2"() -> (w289:bool)
    n178 = Or(x=w289, y=w290) -> (x .or. y?=→"alerte":bool)
    n179 = Number To Decimal String(number=w310) -> (decimal integer string=w301:string)  [unwired: 1 in]
    n180 = call "controle energie.vi"("Date Fin"="Date Fin", "Error in (no error)"=w362, "Date Debut"="Date Debut", "ID compresseur"="ID compresseur", "Connection In"=w381) -> ("Error out"=w344:errorcluster, "Temp"=→"temp de marche en heure":dbl, "Emergie"=w350:dbl, "Connection Out"=w346:refnum<k7>)  [unwired: 3 in]
    "energie consommer kwh" <- w350
    n181 = Concatenate Strings(w301, w298) -> (→"Temps restants C":string)
    n182 = String Subset(string="Prix KWH", length (rest)=3 ("length (rest)")) -> (substring=w352:string)  [unwired: 1 in]
    n183 = Fract/Exp String To Number(string=w352) -> (number=w351:dbl)  [unwired: 3 in, 1 out]
    n184 = Multiply(x=w351, y=w350) -> (x*y=w349:dbl)
    n185 = call "KPI.vi"("Connection In"=w346, "ID compresseur"="ID compresseur", "Date Debut"="Date Debut", "Date Fin"="Date Fin", "Error in (no error)"=w344) -> ("Temps de fonctionnement total"=→"Temps de fonctionnement total":string, "Taux d’utilisation (%)"=→"Taux d’utilisation (%)":string, "Connection Out"=w345:refnum<k7>, "Pression moyenne"=→"Pression moyenne":string, "température moyenne"=→"température moyenne":string, "Nombre de démarrages / arrêts"=→"Nombre de démarrages / arrêts":string, "Temps d'arret total"=→"Temps d'arret total":string, "Error out"=w343:errorcluster)  [unwired: 3 in]
    n186 = Add(x=w361, y=1) -> (x+y=w359:i32)
    n187 = Divide(x=w349, y=1000.0) -> (x/y=→"COUT EN DT":dbl)
    n188 = call "maintenance_check.vi"("Error in (no error)"=w343, "iteration"=w359, "number"="compresseur id", "Connection In"=w345) -> ("Error out"=w292:errorcluster, "Durée de vie du Courroie"=→"Durée de vie du courroie":string, "Nombre d'heure de marche H"=→"Nombre d'heure de marche H":string, "Connection Out"=w291:refnum<k7>, "Nombre d'heure de marche C"=→"Nombre d'heure de marche C":string, "Durée de vie du huile"=→"Durée de vie du huile":string, "Derniére date de changement  C"=→"Derniére date de changement C":string, "Derniére date de changement  H"=→"Derniére date de changement  H":string)
    n189 = Not(x=w317) -> (.not. x?=w316:bool)
  }
  n190 = call <vilib>:"SQL Close.vi"("Connection In"=w11, "Error in (no error)"=w10) -> ("Error out"=→"error out 2":errorcluster)  [unwired: 17 in]
  n191 = call <vilib>:"SQL Close.vi"("Connection In"=w4, "Error in (no error)"=w3) -> ("Error out"=→"Error out 2":errorcluster)  [unwired: 17 in]
